vi "ValidateJog.vi"(8 "error in (no error)":errorcluster, 10 "targetJog":dbl, 11 "KST101 in":refnum<class "KST101.lvclass">) -> (0 "error out":errorcluster, 2 "validJog?":bool, 3 "KST101 out":refnum<class "KST101.lvclass">)   [LabVIEW 2016, in "Stepper Motor Controller.lvlib" / "KST101.lvclass"]
uses:
  KST101.lvclass
  KST101.lvclass/KST101.ctl
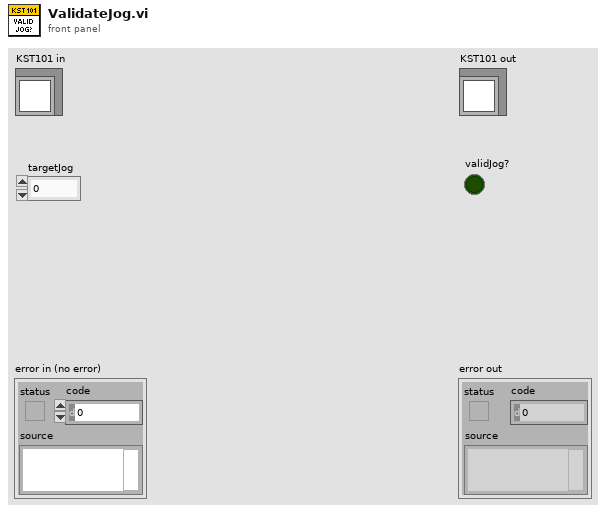
[diagram p1: front panel]
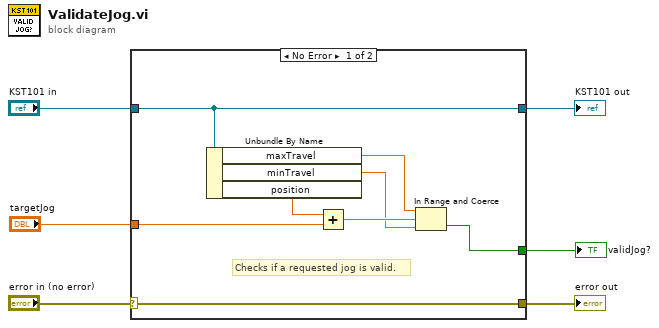
[diagram p0: block diagram]
diagram:
  n1 = case shown="No Error" "error in (no error)" {
    selector: "error in (no error)" -> [w14 w16]
    tunnel: [w14 w16] -> w5
    tunnel: [w13 w15] -> w3
    tunnel: "KST101 in" -> [w13 w15]
    tunnel: "targetJog" -> [w12 _]
    tunnel: [w8 _] -> w1
    frame No Error {
      # "Checks if a requested jog is valid."
      n2 = Unbundle By Name(w13) -> ("maxTravel"=w10:dbl, "minTravel"=w7:dbl, "position"=w11:dbl)
      n3 = Add(x=w11, y=w12) -> (x+y=w9:dbl)
      n4 = In Range and Coerce(upper limit=w10, x=w9, lower limit=w7) -> (In Range?=w8:bool)  [unwired: 1 out]
    }
    frame Error {
    }
  }
  "error out" <- w5
  "KST101 out" <- w3
  "validJog?" <- w1
